vi "drivetrain_globals.vi"() -> ()   [LabVIEW 2011]
uses:
  drivetrain_drive_mode.ctl
  gear_shift_state.ctl
panel:
  in  "peak time":u32=2000
  in  "gear shift state":T1
  in  "Shift Servo Positions (0-1)":dbl[](array[numeric])=[0.25, 0.7, 0.0, 1.0]
  in  "drive mode":T2
  in  "Drivetrain Gains":dbl[](array[numeric])=[0.0, 0.0]
  in  "Drivetrain Speeds":dbl[](array[numeric])=[4.0, 16.5]
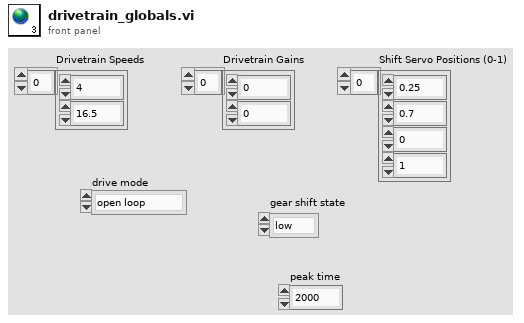
[diagram p1: front panel]
types:
  T1 = typedef "gear_shift_state.ctl" = enum16{"low", "high"}
  T2 = typedef "drivetrain_drive_mode.ctl" = enum16{"open loop", "closed loop"}
diagram:
